vi "Deserialize.vi"(7 "Anything":variant, 8 "error in (no error)":errorcluster, 9 "Deserialize Options":T1, 10 "Serialized Text":string, 11 "BlueSerializer in":refnum<class "BlueSerializer.lvclass">) -> (0 "error out":errorcluster, 2 "Variant":variant, 3 "BlueSerializer out":refnum<class "BlueSerializer.lvclass">)   [LabVIEW 2020, in "BlueSerialization.lvlib" / "BlueSerializer.lvclass"]
doc: "Deserializes a string into any <b>BlueSerializable</b> object\n\nOptions:\n<b>expand objects on type conflict?</b>\nIf True, then the wired object is allowed to be more-specific than the serialized text. The returned object will be the more specific object. If false, then an error will be returned in this situation.\n\n<b>slice flattened object data on error?</b>\nIf True, then the framework will iterate upwards through a class hierarchy until it finds a load-able class instance. This means that the returned data may be less-specific than the serialized text.\n\n<b>sliceable class names</b>\nIf a class isn't found in memory, then the framework will be allowed to slice class names in this list until finding a class in the hierarchy that is load-able.\n\n<b>deserialize non-BlueSerializable objects from hex?</b>\nIf True, then the framework will unflatten non-BlueSerializable objects using the \"unflatten from text\" node. If False, then non-BlueSerializable objects found in the reference data will yield and error.\n\n<b>error on inserted parent levels?</b>\nIf True, then the framework allows for class mutation history where a parent level was added. This means that your output data will contain default-data for this added class layer. If False, then error\n\n<b>error on obsolete parent levels?</b>\nIf True, then the framework allows for class mutation history where a parent level was removed. This means that data for dropped class layers in your serialized text will also be unused. If False, then error.\n\n<b>Preserve wired non-serialized data?</b>\n\"Don't Preserve\": non-serialized data will not be preserved.\n\"Preserve (error on less-specific wired types)\": non-serialized data will be preserved. However, if a wired object is found to be less specific than the serialized object, then you will receive an error.\n\"Preserve (except on less-specific wired types)\": non-serialized data will be preserved except where a wired object is found to be less specific than the serialized object. (It's not possible to preserve data in this situation without class composition.)\n\n<b>Preserve wired serialized data?</b>\nIf True, then the serialized data on the wired object will be preserved prior to being populated by the serialized text input. This is relevant if your object in memory has serializable data fields not present in the serialized text. If false, then default values for the SerializableData will be used."
uses:
  BlueSerializer.lvclass
  DeserializeOptions.ctl
  DeserializeSlicingOptions.ctl
  DeserializeMutationOptions.ctl
  DeserializePreservationOptions.ctl
  PreserveNonWiredDataOption.ctl
  BlueSerializer.lvclass/BlueSerializer.ctl
  ClearClassNameCache.vi
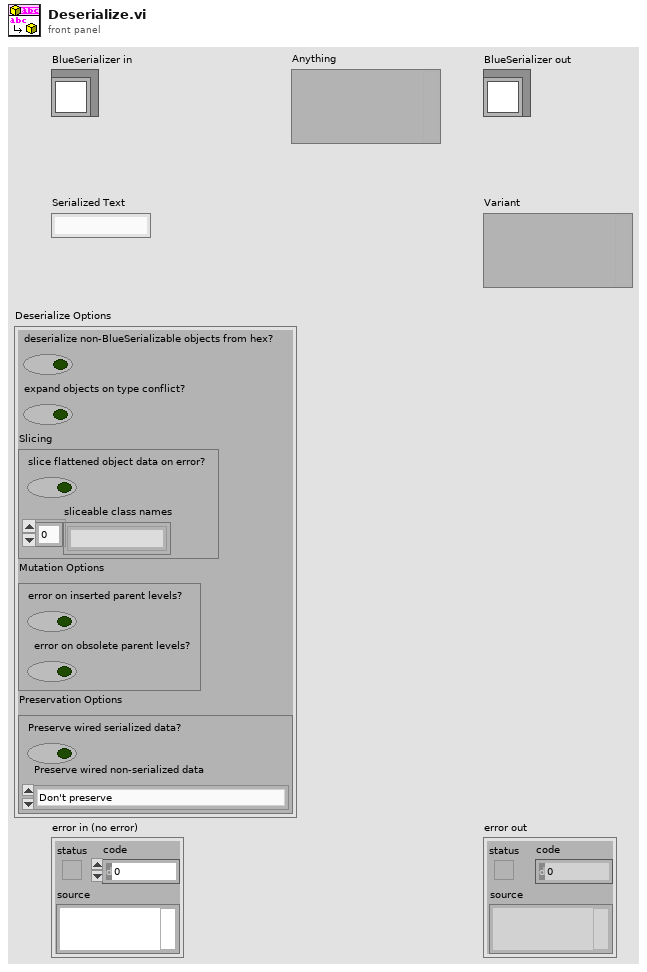
[diagram p1: front panel]
types:
  T1 = typedef "BlueSerialization.lvlib/BlueSerializer.lvclass/DeserializeOptions.ctl" = cluster{"deserialize non-BlueSerializable objects from hex?":bool, "expand objects on type conflict?":bool, "Slicing":T2, "Mutation Options":T3, "Preservation Options":T4}
  T2 = typedef "BlueSerialization.lvlib/BlueSerializer.lvclass/DeserializeSlicingOptions.ctl" = cluster{"slice flattened object data on error?":bool, "sliceable class names":string[]}
  T3 = typedef "BlueSerialization.lvlib/BlueSerializer.lvclass/DeserializeMutationOptions.ctl" = cluster{"error on inserted parent levels?":bool, "\terror on obsolete parent levels?":bool}
  T4 = typedef "BlueSerialization.lvlib/BlueSerializer.lvclass/DeserializePreservationOptions.ctl" = cluster{"Preserve wired serialized data?":bool, "Preserve wired non-serialized data":T5}
  T5 = typedef "BlueSerialization.lvlib/BlueSerializer.lvclass/PreserveNonWiredDataOption.ctl" = enum16{"Don't preserve", "Preserve (error on less-specific wired types)", "Preserve (except on less-specific wired types)"}
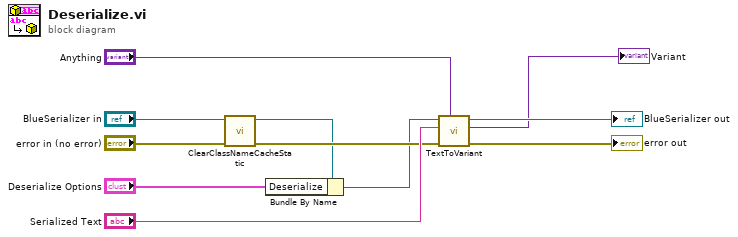
[diagram p0: block diagram]
diagram:
  n1 = call "ClearClassNameCacheStatic.vi"("error in (no error)"="error in (no error)", "BlueSerializer in"="BlueSerializer in") -> ("error out"=w4:errorcluster, "BlueSerializer out"=w3:refnum<class "BlueSerializer.lvclass">)  [unwired: 8 in]
  n2 = Bundle By Name(cluster=w3, "Deserialize"="Deserialize Options") -> (w1:refnum<class "BlueSerializer.lvclass">)
  n3 = call-dynamic "TextToVariant.vi"("Data Type"="Anything", "error in (no error)"=w4, "Serializable Text"="Serialized Text", "BlueSerializer in"=w1) -> ("error out"=→"error out":errorcluster, "Variant out"=→"Variant":variant, "BlueSerializer out"=→"BlueSerializer out":refnum<class "BlueSerializer.lvclass">)  [unwired: 5 in]
